vi "DAC Save Results.vi"(8 "error in":errorcluster, 9 "Log Details?":bool, 10 "tdms file":refnum<k34>, 11 "DAC Inclino in":refnum<class "DAC Inclinometer.lvclass">) -> (0 "error out":errorcluster)   [LabVIEW 2019, in "DAC.lvlib" / "DAC Inclinometer.lvclass"]
uses:
  DAC Inclinometer.lvclass
  DAC.lvclass
  C:/Users/wg/Documents/LV_Projects/test-stand/App/DAC/DAC.lvclass
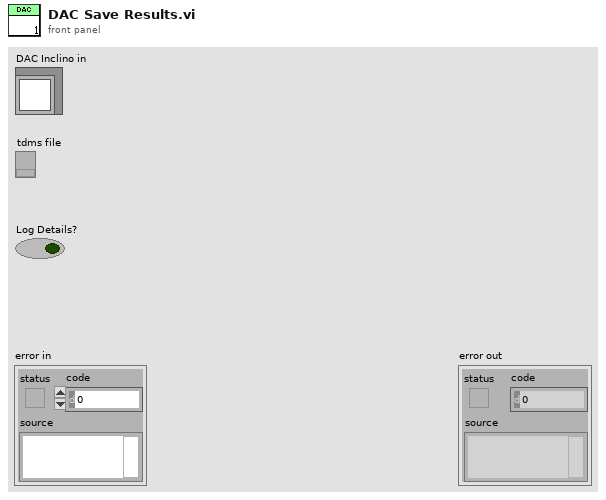
[diagram p1: front panel]
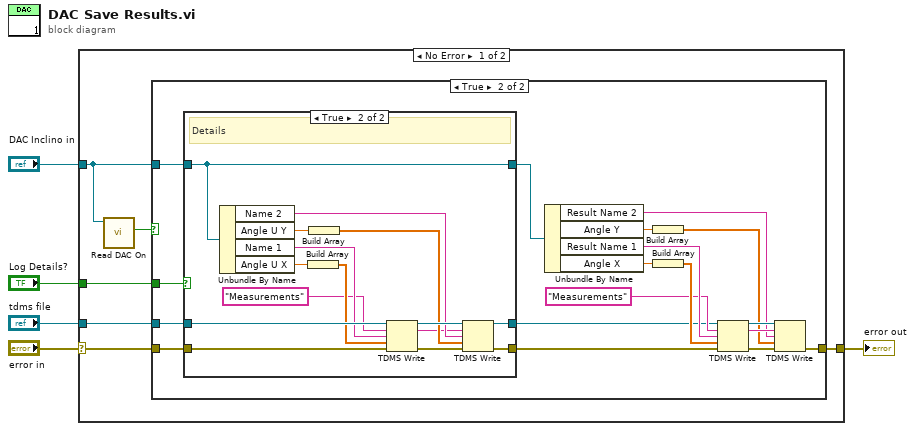
[diagram p0: block diagram]
diagram:
  n1 = case shown="No Error" "error in" {
    selector: "error in" -> [w8 w49]
    tunnel: "DAC Inclino in" -> [w11 _]
    tunnel: "tdms file" -> [w9 _]
    tunnel: [w7 w49] -> w3
    tunnel: "Log Details?" -> [w6 _]
    frame No Error {
      n2 = call "Read DAC On.vi"("DAC in"=w11) -> ("DAC On"=w10:bool)  [unwired: 8 in, 2 out]
      n3 = case shown="True" w10 {
        tunnel: w11 -> [_ w26]
        tunnel: w9 -> [_ w24]
        tunnel: w8 -> [w12 w23]
        tunnel: [w12 w13] -> w7
        tunnel: w6 -> [_ w25]
        frame False {
        }
        frame True {
          n4 = case shown="True" w25 {
            tunnel: w24 -> [w32 w48]
            tunnel: w23 -> [w33 w44]
            tunnel: w26 -> [w31 w43]
            tunnel: [w33 w35] -> w19
            tunnel: [w32 w36] -> w20
            tunnel: [w31 w43] -> w22
            frame False {
            }
            frame True {
              # "Details"
              n5 = Unbundle By Name(w43) -> ("Name 2"=w38:string, "Angle U Y"=w42:dbl, "Name 1"=w45:string, "Angle U X"=w47:dbl)
              n6 = Build Array(w47) -> (w46:dbl[])
              n7 = Build Array(w42) -> (w39:dbl[])
              n8 = TDMS Write(0:w48, 5:"Measurements" ("group name in (Untitled)"), 7:w45, 9:w46, 11:w44) -> (4:w41:refnum<k34>, 6:w34:string, 15:w40:errorcluster)  [unwired: 1 in, 1 out]
              n9 = TDMS Write(0:w41, 5:w34, 7:w38, 9:w39, 11:w40) -> (4:w36:refnum<k34>, 15:w35:errorcluster)  [unwired: 1 in, 2 out]
            }
          }
          n10 = Unbundle By Name(w22) -> ("Result Name 2"=w14:string, "Angle Y"=w21:dbl, "Result Name 1"=w28:string, "Angle X"=w30:dbl)
          n11 = Build Array(w21) -> (w15:dbl[])
          n12 = Build Array(w30) -> (w29:dbl[])
          n13 = TDMS Write(0:w20, 5:"Measurements" ("group name in (Untitled)"), 7:w28, 9:w29, 11:w19) -> (4:w18:refnum<k34>, 6:w17:string, 15:w16:errorcluster)  [unwired: 1 in, 1 out]
          n14 = TDMS Write(0:w18, 5:w17, 7:w14, 9:w15, 11:w16) -> (15:w13:errorcluster)  [unwired: 1 in, 3 out]
        }
      }
    }
    frame Error {
    }
  }
  "error out" <- w3
